vi "ClawGlobal.vi"() -> ()   [LabVIEW 2023]
panel:
  in  "ClawAmps":dbl
  out "HasCube":bool
  out "HasCone":bool
  in  "SonarDist":dbl
  in  "ClawDemand":dbl
  out "ClawOpen?":bool
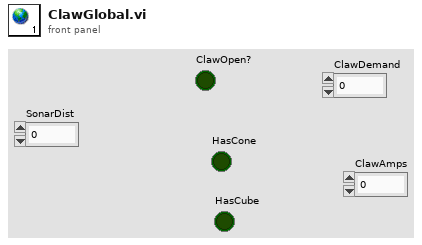
[diagram p1: front panel]
diagram:
